vi "roboRIO v1.0 Write RSL.vi"(8 "error in (no error)":errorcluster, 9 "bool Value List":bool[](array[boolean]), 10 "Channel List":T3, 11 "myRIO Ref In":T1) -> (0 "error out":errorcluster, 3 "myRIO Ref Out":T1)   [LabVIEW 2021]
uses:
  <vilib>/myRIO/Common/Instrument Driver Framework/roboRIO v1.0/RSL/typedefs/RSL Channels List.ctl
  <vilib>/myRIO/Common/Instrument Driver Framework/roboRIO v1.0/RSL/typedefs/RSL Channels Enum.ctl
  <vilib>/myRIO/Common/Instrument Driver Framework/Utilities/typedefs/myRIO v1.0 Reference.ctl
  <vilib>/myRIO/Common/Instrument Driver Framework/Utilities/typedefs/Generic FPGA Reference.ctl
  <vilib>/myRIO/Common/Instrument Driver Framework/roboRIO v1.0/RSL/typedefs/RSL FPGA Reference.ctl
  <vilib>/rvi/errors/niLvFpgaAdjustHostInterfaceError.vi
  <vilib>/rvi/interface/nirviReadWriteControl/nirviReadWriteControl.xnode
  <vilib>/rvi/interface/Simulation/niFpgaSimulationCallBeginRW.vi
  NiFpgaLv.dll
panel:
  # "This VI writes boolean values to a user specified a list of DIO channels on the myRIO v1.0 hardware. The value is input as a boolean value. Please see Block Diagram for details."
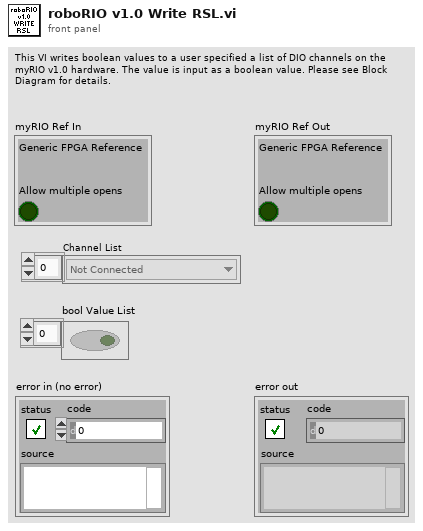
[diagram p1: front panel]
types:
  T1 = typedef "myRIO v1.0 Reference.ctl" = cluster{"Generic FPGA Reference":T2, "Allow multiple opens":bool}
  T2 = typedef "Generic FPGA Reference.ctl" = refnum<k20>
  T3 = typedef "RSL Channels List.ctl" = T4[]
  T4 = typedef "RSL Channels Enum.ctl" = enum16{"Not Connected", "RSL/RSL0"}
  T5 = typedef "RSL FPGA Reference.ctl" = refnum<k20>
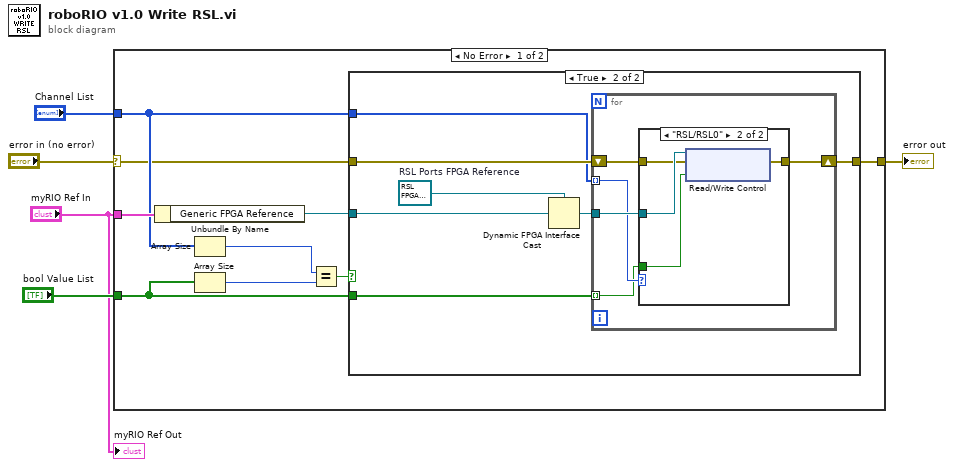
[diagram p0: block diagram]
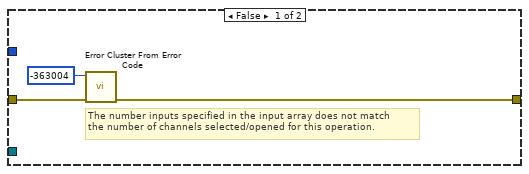
[diagram p2: hidden frame]
diagram:
  n1 = case shown="No Error" "error in (no error)" {
    selector: "error in (no error)" -> [w7 w35]
    tunnel: "myRIO Ref In" -> [w14 _]
    tunnel: [w13 w35] -> w4
    tunnel: "Channel List" -> [w10 _]
    tunnel: "bool Value List" -> [w9 _]
    frame No Error {
      n2 = Unbundle By Name(w14) -> ("Generic FPGA Reference"=w6:T2)
      n3 = Array Size(array=w10) -> (size(s)=w12:i32)
      n4 = Array Size(array=w9) -> (size(s)=w11:i32)
      n5 = Equal?(x=w12, y=w11) -> (x = y?=w8:bool)
      n6 = case shown="True" w8 {
        tunnel: w10 -> [_ w19]
        tunnel: w9 -> [_ w18]
        tunnel: w6 -> [_ w23]
        tunnel: w7 -> [w16 w21]
        tunnel: [w15 w20] -> w13
        frame False {
          # "The number inputs specified in the input array does not match\nthe number of channels selected/opened for this operation."
          n7 = call <vilib>:"Error Cluster From Error Code.vi"("error in (no error)"=w16, "error code (0)"=-363004) -> ("error out"=w15:errorcluster)  [unwired: 7 in]
        }
        frame True {
          w24 = T5 refnum  # RSL Ports FPGA Reference
          n8 = Dynamic FPGA Interface Cast(Session In=w24, Type=w23) -> (Session Out=w22:T5)
          n9 = for {
            tunnel: w22 -> [w29]
            tunnel: w19 -> [w26] mode=indexing
            shift-right: [w27] -> w20
            shift-left: w21 -> [w28]
            tunnel: w18 -> [w25] mode=indexing
            n10 = case shown="\"RSL/RSL0\"" w26 {
              tunnel: w29 -> [_ w33]
              tunnel: w28 -> [w30 w32]
              tunnel: [w30 w34] -> w27
              tunnel: w25 -> [_ w31]
              frame "Not Connected", Default {
              }
              frame "RSL/RSL0" {
                n11 = xnode "Read/Write Control"("FPGA VI Reference In"=w33, "error in"=w32, "DO.RSL.OUT"=w31) -> ("error out"=w34:errorcluster)  [unwired: 1 out]
              }
            }
          }
        }
      }
    }
    frame Error {
    }
  }
  "error out" <- w4
  "myRIO Ref Out" <- "myRIO Ref In"
